vi "Game_simpleError.vi"(7 "command":string, 8 "error in (no error)":errorcluster, 11 "Queue Bus":T1) -> (0 "error out":errorcluster, 3 "Queue Bus OUT":T1)   [LabVIEW 2020]
uses:
  Typedefs/queueBus.ctl
  Typedefs/communicationData.ctl
panel:
  out "code":i32
  out "source":string
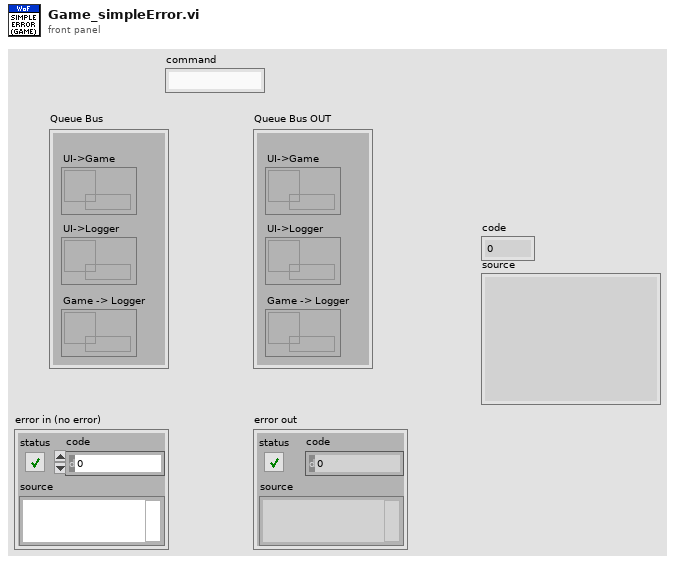
[diagram p1: front panel]
types:
  T1 = typedef "queueBus.ctl" = cluster{"UI->Game":refnum<queue>, "UI->Logger":refnum<queue>, "Game -> Logger":refnum<queue>}
  T2 = typedef "communicationData.ctl" = cluster{"command":string, "payload":variant, "response":variant}
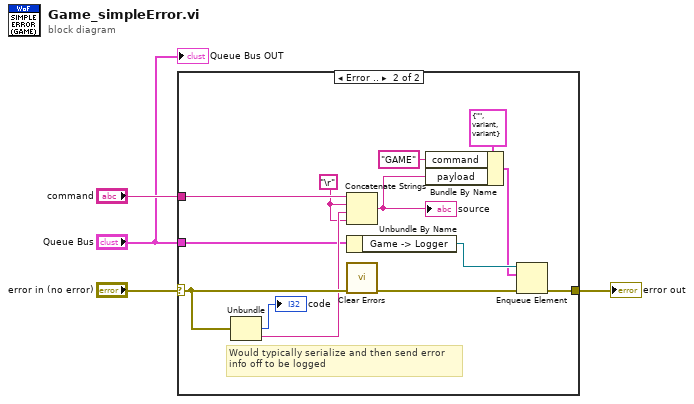
[diagram p0: block diagram]
diagram:
  n1 = case shown="Error .." "error in (no error)" {
    selector: "error in (no error)" -> [w5 w17]
    tunnel: [w5 w12] -> w3
    tunnel: "command" -> [_ w15]
    tunnel: "Queue Bus" -> [_ w11]
    frame No Error {
    }
    frame Error {
      w13 = "\r"
      # "Would typically serialize and then send error\ninfo off to be logged"
      n2 = Unbundle(w17) -> ("code"=→"code":i32, "source"=w14:string)  [unwired: 1 out]
      n3 = Concatenate Strings(w15, w13, w14, w13) -> (w8:string)
      "source" <- w8
      n4 = Unbundle By Name(w11) -> ("Game -> Logger"=w7:refnum<queue>)
      n5 = call <vilib>:"Clear Errors.vi"("error in (no error)"=w17) -> ("error out"=w18:errorcluster)  [unwired: 5 in, 1 out]
      n6 = Bundle By Name(cluster=T2 {"command"="", "payload"=variant, "response"=variant} ("communication"), "command"="GAME", "payload"=w8) -> (w6:T2)
      n7 = Enqueue Element(queue=w7, element=w6, error in (no error)=w18) -> (error out=w12:errorcluster)  [unwired: 1 in, 2 out]
    }
  }
  "error out" <- w3
  "Queue Bus OUT" <- "Queue Bus"
